vi "Goal Manager.vi"(8 "error in (no error)":errorcluster, 10 "SQL Date":string, 11 "Database.lvclass":refnum<class "Database.lvclass">) -> (0 "error out":errorcluster, 3 "Database.lvclass":refnum<class "Database.lvclass">)   [LabVIEW 2018]
uses:
  support/classes/database/Database.lvclass
  support/classes/Category/Category.lvclass
panel:
  in  "Add":bool
  in  "Done":bool
  in  "Goal Amount":dbl
  in  "Category Table":i32(listbox)
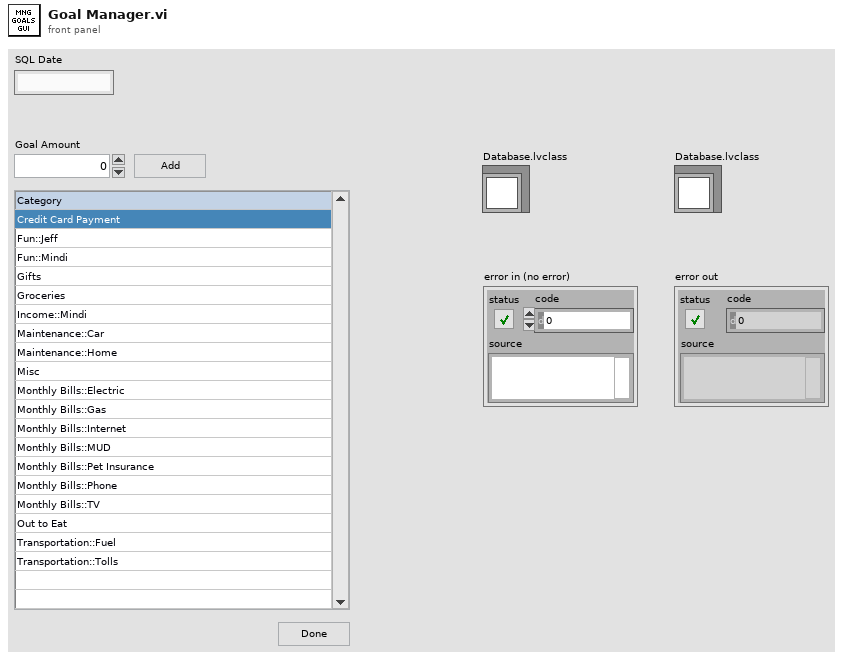
[diagram p1: front panel]
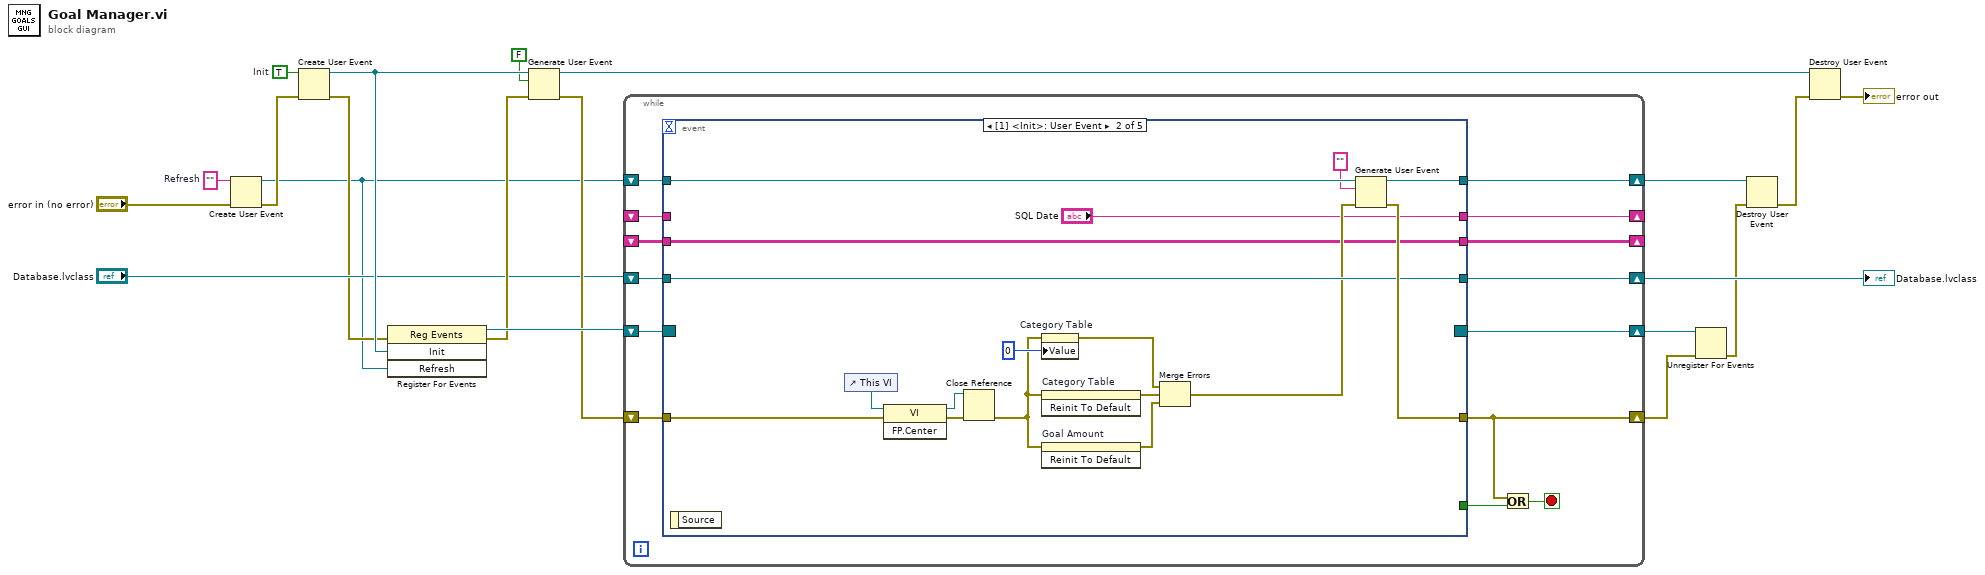
[diagram p0: block diagram]
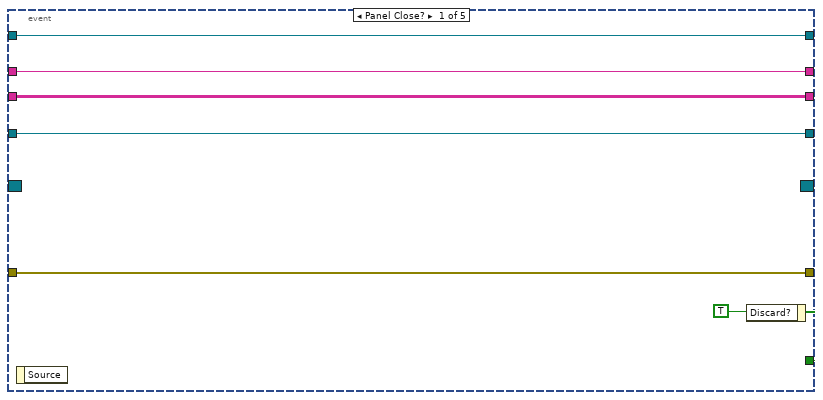
[diagram p2: hidden frame]
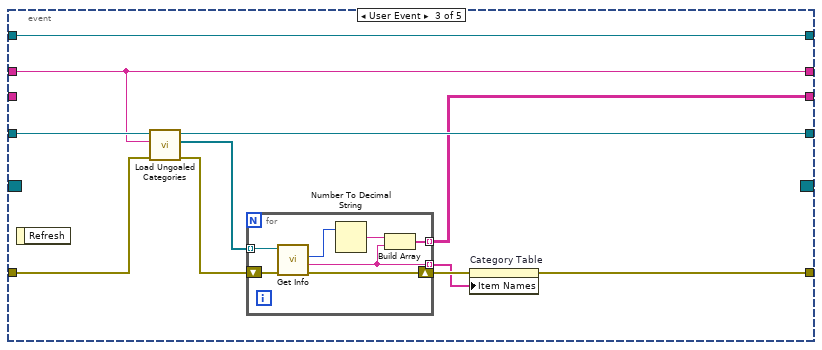
[diagram p3: hidden frame]
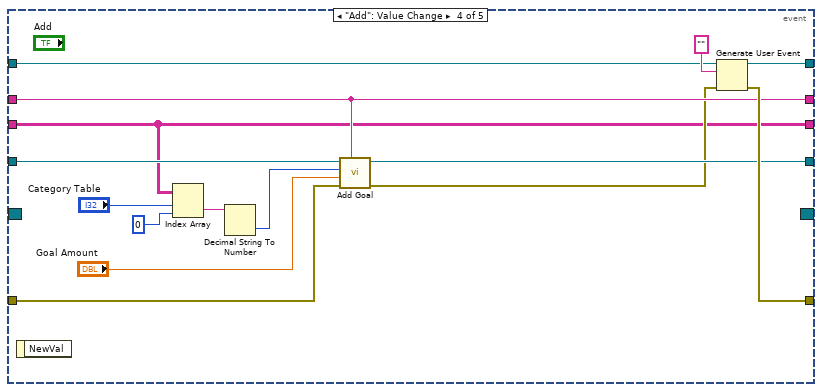
[diagram p4: hidden frame]
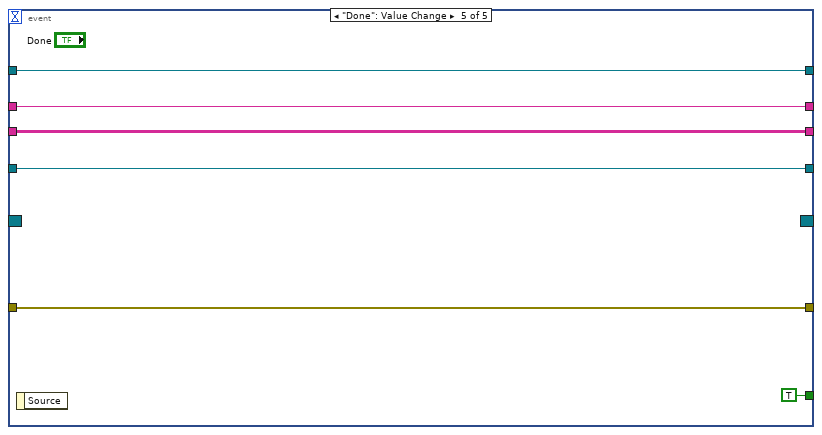
[diagram p5: hidden frame]
diagram:
  w1 = ""  # Refresh
  w20 = TRUE  # Init
  n1 = Create User Event(user event datatype=w1, error in="error in (no error)") -> (user event=w2:refnum<user-event>, error out=w4:errorcluster)
  n2 = Create User Event(user event datatype=w20, error in=w4) -> (user event=w18:refnum<user-event>, error out=w12:errorcluster)
  n3 = register-events(error in=w12, w18, w2) -> (reference out=w19:refnum<event-registration>, error out=w17:errorcluster)  [unwired: 1 in]
  n4 = Generate User Event(user event=w18, event data cluster=FALSE ("event data"), error in=w17) -> (user event out=w11:refnum<user-event>, error out=w16:errorcluster)  [unwired: 1 in]
  n5 = while {
    shift-right: [w32] -> w9
    shift-left: w19 -> [w34]
    shift-right: [w31] -> w8
    shift-left: w16 -> [w33]
    shift-right: [w27] -> w13
    shift-left: "Database.lvclass" -> [w28]
    shift-right: [w25] -> w5
    shift-left: w2 -> [w26]
    shift-right: [w24] -> _
    shift-left: _ -> [w23]
    shift-right: [w22] -> _
    shift-left: _ -> [w21]
    stop <- w29 stop-if-true
    n6 = event shown="[1] <Init>: User Event" {
      selector: w34 -> [_ _ _ _ _]
      dyn-events: [_ _ _ _ _] -> w32
      timeout: _ -> [_ _ _ _ _]
      tunnel: [w40 _ _ _ TRUE ("Discard?")] -> w30
      tunnel: w33 -> [w39 w53 w64 w83 w93]
      tunnel: [w39 w46 w66 w87 w93] -> w31
      tunnel: w28 -> [w38 w44 w65 w86 w94]
      tunnel: [w38 w44 w62 w84 w94] -> w27
      tunnel: w26 -> [w36 w48 w68 w88 w95]
      tunnel: [w36 w47 w68 w89 w95] -> w25
      tunnel: [w37 "SQL Date" w60 w85 w92] -> w24
      tunnel: w23 -> [w37 _ w60 w85 w92]
      tunnel: [w35 w41 w59 w80 w91] -> w22
      tunnel: w21 -> [w35 w41 _ w80 w91]
      event Panel Close? {
        w40 = TRUE ("Discard?")
        n7 = event-data() -> ()  [unwired: 1 in, 1 out]
        n8 = event-data("Discard?"=w40) -> ()  [unwired: 1 in, 1 out]
      }
      event User Event {
        n9 = event-data() -> ()  [unwired: 1 in, 1 out]
        n10 = control-ref of="This VI"() -> (w54:refnum<vi>)
        n11 = invoke class="VI" method="FP.Center"(reference=w54, error in=w53) -> (reference out=w51:refnum<vi>, error out=w52:errorcluster)  [unwired: 1 in, 1 out]
        n12 = Close Reference(reference=w51, error in (no error)=w52) -> (error out=w50:errorcluster)
        n13 = property on="Category Table" class="LstBox (strict)"(error in=w50, "Value"=0 ("Category Table")) -> (error out=w49:errorcluster)  [unwired: 1 in, 1 out]
        n14 = invoke on="Category Table" class="LstBox (strict)" method="Reinit To Default"(error in=w50) -> (error out=w56:errorcluster)  [unwired: 2 in, 2 out]
        n15 = invoke on="Goal Amount" class="DigNum (strict)" method="Reinit To Default"(error in=w50) -> (error out=w57:errorcluster)  [unwired: 2 in, 2 out]
        n16 = Merge Errors(w49, w56, w57) -> (w43:errorcluster)
        n17 = Generate User Event(user event=w48, event data cluster="" ("event data"), error in=w43) -> (user event out=w47:refnum<user-event>, error out=w46:errorcluster)  [unwired: 1 in]
      }
      event User Event {
        n18 = event-data() -> ()  [unwired: 1 in, 1 out]
        n19 = call "Load Ungoaled Categories.vi"("error in (no error)"=w64, "SQL Date"=w60, "Database in"=w65) -> ("error out"=w63:errorcluster, "Categories with No Goal"=w61:refnum<class "Category.lvclass">[], "Database out"=w62:refnum<class "Database.lvclass">)  [unwired: 6 in]
        n20 = for {
          shift-right: [w75] -> w67
          shift-left: w63 -> [w74]
          tunnel: w61 -> [w73] mode=indexing
          tunnel: [w70] -> w59 mode=indexing
          tunnel: [w69] -> w58 mode=indexing
          n21 = call "Get Info.vi"("error in (no error)"=w74, "Category in"=w73) -> ("error out"=w75:errorcluster, "Name"=w69:string, "id"=w72:i32)  [unwired: 6 in, 1 out]
          n22 = Number To Decimal String(number=w72) -> (decimal integer string=w71:string)  [unwired: 1 in]
          n23 = Build Array(w71, w69) -> (w70:string[])
        }
        n24 = property on="Category Table" class="LstBox (strict)"(error in=w67, "Item Names"=w58) -> (error out=w66:errorcluster)  [unwired: 1 in, 1 out]
      }
      event "Add": Value Change {
        n25 = event-data() -> ()  [unwired: 1 in, 1 out]
        n26 = Index Array(array=w80, index (row)="Category Table", index (col)=0 ("disabled index (col)")) -> (element=w78:string)
        n27 = Decimal String To Number(string=w78) -> (number=w77:i32)  [unwired: 2 in, 1 out]
        n28 = call "Add Goal.vi"("SQL Date"=w85, "error in (no error)"=w83, "Goal Amount"="Goal Amount", "Category_id"=w77, "Database in"=w86) -> ("error out"=w82:errorcluster, "Database out"=w84:refnum<class "Database.lvclass">)  [unwired: 5 in]
        n29 = Generate User Event(user event=w88, event data cluster="" ("event data"), error in=w82) -> (user event out=w89:refnum<user-event>, error out=w87:errorcluster)  [unwired: 1 in]
      }
      event "Done": Value Change {
        n30 = event-data() -> ()  [unwired: 1 in, 1 out]
      }
    }
    n31 = Or(x=w31, y=w30) -> (x .or. y?=w29:bool)
  }
  "Database.lvclass" <- w13
  n32 = Unregister For Events(event registration refnum=w9, error in=w8) -> (error out=w10:errorcluster)
  n33 = Destroy User Event(user event=w5, error in=w10) -> (error out=w7:errorcluster)
  n34 = Destroy User Event(user event=w11, error in=w7) -> (error out=→"error out":errorcluster)
